vi "InstrumentSetup.vi"() -> ()   [LabVIEW 2018, in "InstrControl.lvclass"]
uses:
  InstrControl.lvclass
  ArduinoControl/ArduinoControl.lvclass
  Switching/Switching.lvclass
panel:
  in  "PXI/LXI Switching":T1={"MUX "="12", "Matrix"="13", "Breadboard"="14", "MUX  PN"="40-635-108", "Matrix PN"="40-332-002", "Breadboard PN"="40-220A-501-S6"}
  in  "Keithley 2657A Configurations":cluster{"Current Limit":sgl}={"Current Limit"=1e-05}
  in  "Keithley 487_2 Configurations":cluster{"Compliance":u16, "Range:":u16} {"Range:" items=["Autorange", "2nA", "20nA", "200nA", "2 microAmp", "20 microAmp", "200 microAmp", "2 milliAmp"]; "Compliance" items=["20µA", "2mA"]}
  in  "Instrument GPIB addresses":T2={"KE 2410"={"Instrument name"="Keithley 2410", "GPIB address"="1:24", "Instrument type"=0}, "KE 6517"={"Instrument name"="Keithley 6517", "GPIB address"="27", "Instrument type"=0}, "KE 487"={"Instrument name"="Keithley 487", "GPIB address"="22", "Instrument type"=0}, "KE 2657A"={"Instrument name"="Keithley 2657A", "GPIB address"="2:16", "Instrument type"=0}, "KE 236"={"Instrument name"="Keithley 236", "GPIB address"="16", "Instrument type"=0}, "WK 6440B"={"Instrument name"="WayneKerr 6440B", "GPIB address"="0:6", "Instrument type"=1}, "WK 6425"={"Instrument name"="WayneKerr 6425", "GPIB address"="17", "Instrument type"=1}, "Pickering Matrix"={"Instrument name"="Pickering Matrix", "GPIB address"="10", "Instrument type"=2}, "KE 2000"={"Instrument name"="Keithley 2000", "GPIB address"="19", "Instrument type"=3}} {"KE 2000"."Instrument type" items=["Supply", "LCR", "Switching", "Multimeter"]; "Pickering Matrix"."Instrument type" items=["Supply", "LCR", "Switching", "Multimeter"]; "WK 6425"."Instrument type" items=["Supply", "LCR", "Switching", "Multimeter"]; "WK 6440B"."Instrument type" items=["Supply", "LCR", "Switching", "Multimeter"]; "KE 236"."Instrument type" items=["Supply", "LCR", "Switching", "Multimeter"]; "KE 2657A"."Instrument type" items=["Supply", "LCR", "Switching", "Multimeter"]; "KE 487"."Instrument type" items=["Supply", "LCR", "Switching", "Multimeter"]; "KE 6517"."Instrument type" items=["Supply", "LCR", "Switching", "Multimeter"]; "KE 2410"."Instrument type" items=["Supply", "LCR", "Switching", "Multimeter"]}
  in  "WayneKerr 6425 Configurations":T3={"RC Configuration"=0, "AC amplitude [V]"=0.1, "AC frequency [Hz]"=1000} {"RC Configuration" items=["serial", "parallel"]}
  in  "MUX & Matrix Configurations":T4={"Matrix address"="1", "Mux1 address"="4", "Mux2 address"="5", "Matrix used?"=TRUE, "Switching"=refnum, "Matrix X Channels"={"Bias Supply / SMU LO"=5, "Bias Supply / SMU HI"=6, "CV Box LO"=3, "CV Box HI"=4, "CV Box LO IN"=7, "CV Box HI IN"=8, "Volt meter LO"=1, "Volt meter HI"=2, "Mux1 C1"=9, "Mux1 C2"=10, "Mux2 C1"=11, "Mux2 C2"=12}}
  in  "WayneKerr 6440B Configurations":T3={"RC Configuration"=0, "AC amplitude [V]"=0.1, "AC frequency [Hz]"=1000} {"RC Configuration" items=["serial", "parallel"]}
  in  "Keithley 2000 Configurations":T5={"Range"=0, "Range Value"=100.0, "Function"=3} {"Function" items=["AC Current", "DC Current", "AC Voltage", "DC Voltage", "2W-Resistance", "4W-Resistance", "Period", "Frequency", "Temperature", "Diode", "Continuity"]; "Range Value" format="%#.2g"; "Range" items=["Auto", "Manual"]}
  in  "Arduino Configuration":T6={"VISA address"="COM3", "T sensor"=enum."SHT", "Arduino"=refnum}
  in  "Keithley 487 Configurations":cluster{"Compliance":u16, "Range:":u16} {"Range:" items=["Autorange", "2nA", "20nA", "200nA", "2 microAmp", "20 microAmp", "200 microAmp", "2 milliAmp"]; "Compliance" items=["20µA", "2mA"]}
  in  "Keithley 2410 Configurations":cluster{"Current Limit":sgl}={"Current Limit"=1e-05}
  in  "Keithley 6517 Configurations":cluster{"Current Limit":u16}={"Current Limit"=1} {"Current Limit" items=["OFF", "ON"]}
  in  "Keithley 236 Configurations":T7={"current \ncompliance level"=0.0001, "compliance/\nmeasurement range (auto:0)"=6} {"compliance/\nmeasurement range (auto:0)" items=["auto / auto", "1 nA / 1.1 V", "10 nA / 11 V", "100 nA / 110 V", "0.001 mA / 110 V", "0.01 mA / 110 V", "0.1 mA / 110 V", "1 mA / 110 V", "10 mA / 110 V", "100 mA / 110 V"]; "current \ncompliance level" format="%.4f"}
  in  "Default GPIB addresses":T8={"KE 487"="22", "KE 6517"="27", "WK 6425"="17", "KE 236"="16", "HP 4263B"="18", "KE 2000"="19", "KE 2410"="1:24", "WK 6440B"="0:6", "Matrix"="10", "KE 2657A"="2:16"}
  # "DEFAULT VALUES FOR INSTRUMENT SETUP"
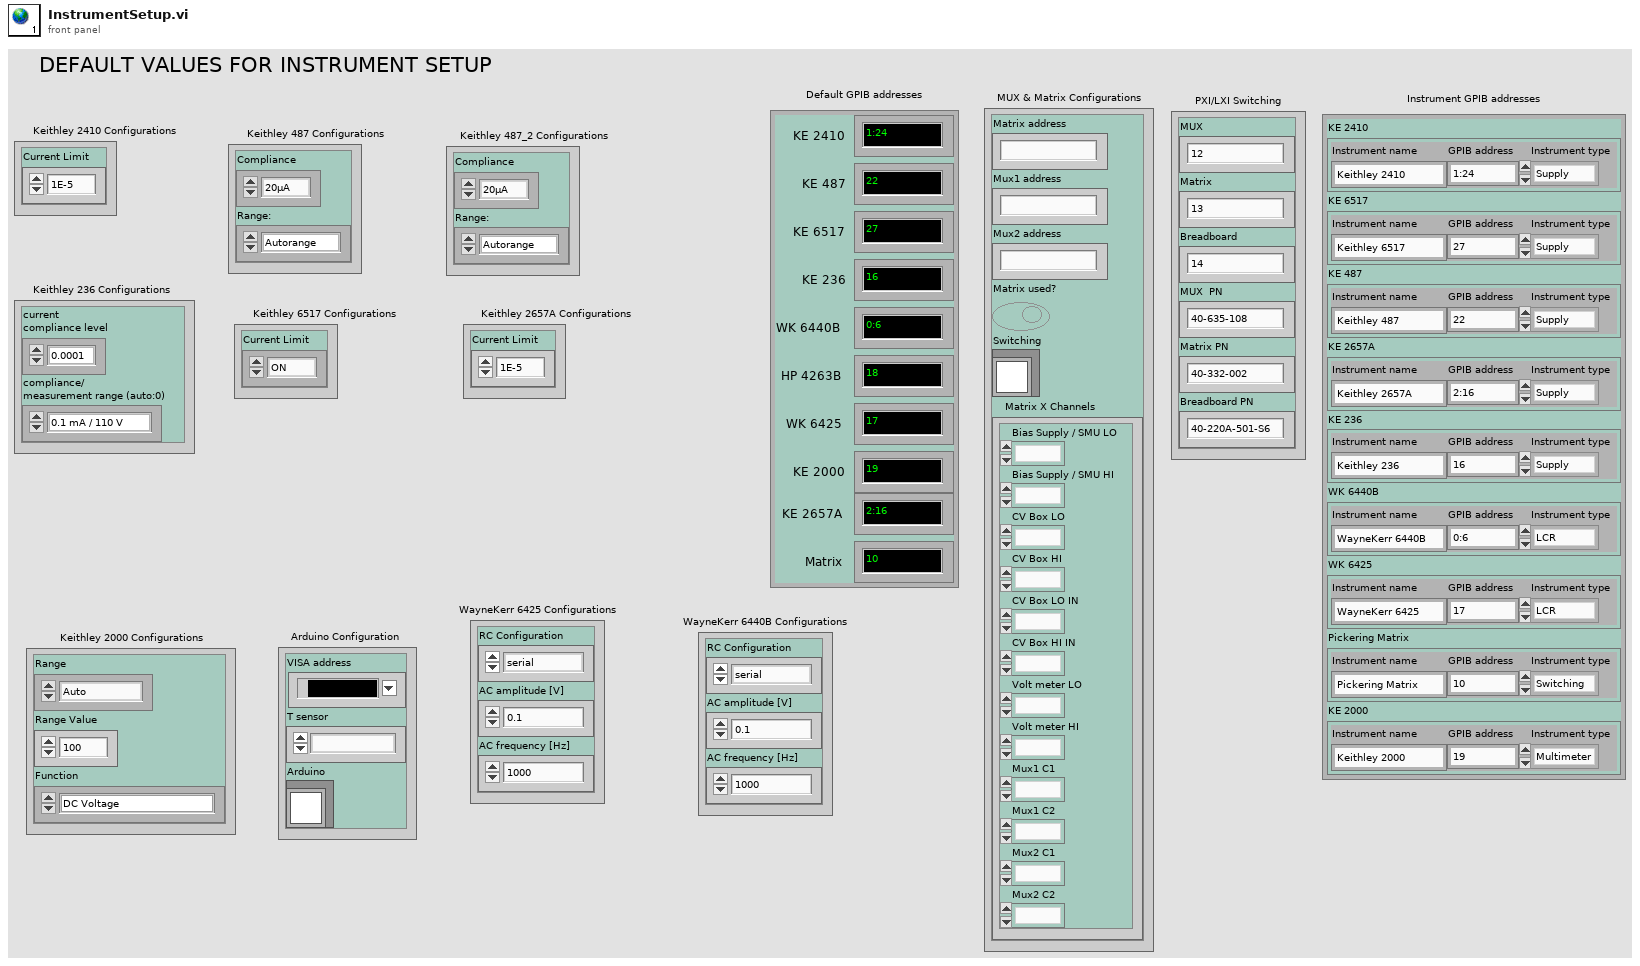
[diagram p1: front panel]
types:
  T1 = cluster{"MUX ":string, "Matrix":string, "Breadboard":string, "MUX  PN":string, "Matrix PN":string, "Breadboard PN":string}
  T2 = cluster{"KE 2410":cluster{"Instrument name":string, "GPIB address":string, "Instrument type":u16}, "KE 6517":cluster{"Instrument name":string, "GPIB address":string, "Instrument type":u16}, "KE 487":cluster{"Instrument name":string, "GPIB address":string, "Instrument type":u16}, "KE 2657A":cluster{"Instrument name":string, "GPIB address":string, "Instrument type":u16}, "KE 236":cluster{"Instrument name":string, "GPIB address":string, "Instrument type":u16}, "WK 6440B":cluster{"Instrument name":string, "GPIB address":string, "Instrument type":u16}, "WK 6425":cluster{"Instrument name":string, "GPIB address":string, "Instrument type":u16}, "Pickering Matrix":cluster{"Instrument name":string, "GPIB address":string, "Instrument type":u16}, "KE 2000":cluster{"Instrument name":string, "GPIB address":string, "Instrument type":u16}}
  T3 = cluster{"RC Configuration":u16, "AC amplitude [V]":dbl, "AC frequency [Hz]":i32}
  T4 = cluster{"Matrix address":string, "Mux1 address":string, "Mux2 address":string, "Matrix used?":bool, "Switching":refnum<class "Switching.lvclass">, "Matrix X Channels":cluster{"Bias Supply / SMU LO":i32, "Bias Supply / SMU HI":i32, "CV Box LO":i32, "CV Box HI":i32, "CV Box LO IN":i32, "CV Box HI IN":i32, "Volt meter LO":i32, "Volt meter HI":i32, "Mux1 C1":i32, "Mux1 C2":i32, "Mux2 C1":i32, "Mux2 C2":i32}}
  T5 = cluster{"Range":u16, "Range Value":dbl, "Function":u16}
  T6 = cluster{"VISA address":refnum<visa-resource-name>, "T sensor":enum16{"SHT", "DS"}, "Arduino":refnum<class "ArduinoControl.lvclass">}
  T7 = cluster{"current \ncompliance level":dbl, "compliance/\nmeasurement range (auto:0)":u16}
  T8 = cluster{"KE 487":string, "KE 6517":string, "WK 6425":string, "KE 236":string, "HP 4263B":string, "KE 2000":string, "KE 2410":string, "WK 6440B":string, "Matrix":string, "KE 2657A":string}
diagram:
